vi "LightSensor.vi"() -> ()   [LabVIEW 2024]
uses:
  Driver/CTIPicoVISA.lvlib
panel:
  out "Identity":T1
  out "Value":u16(graph)
  in  "GroveConnector":enum16{"A0", "A1", "A2"}(ring)
  in  "stop":bool
  in  "VISA resource name in":refnum<visa-resource-name>="COM7"
  out "error out":errorcluster
  # "https://wiki.seeedstudio.com/Grove-Light_Sensor/#upgradable-to-industrial-sensors"
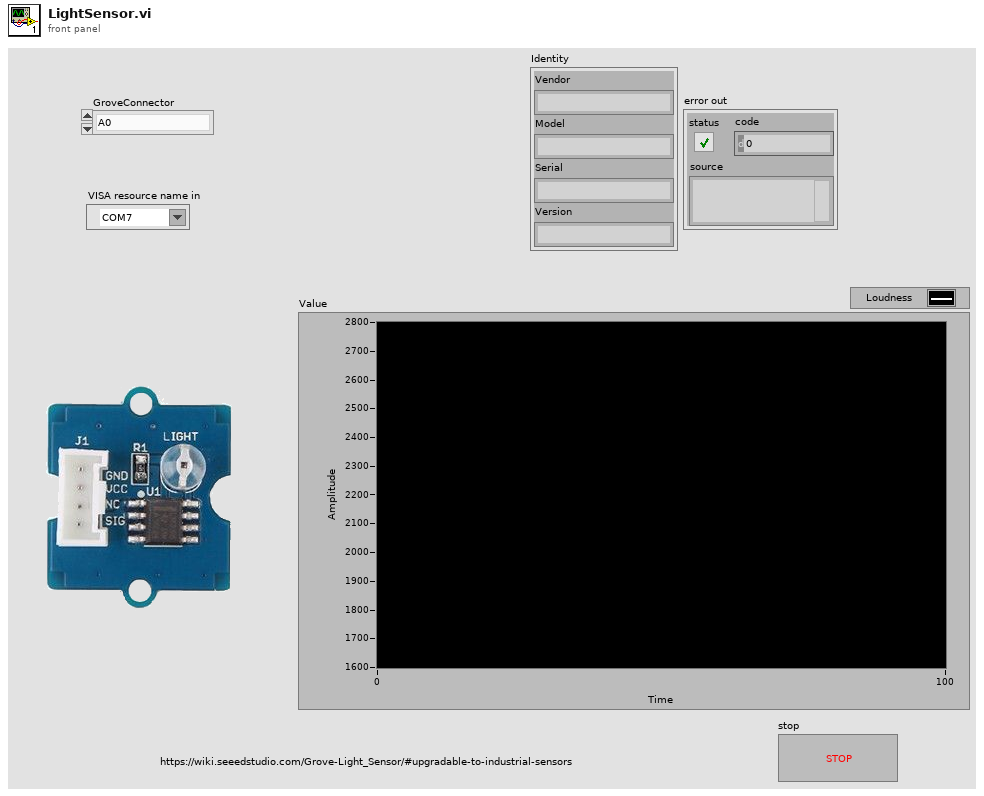
[diagram p1: front panel]
types:
  T1 = cluster{"Vendor":string, "Model":string, "Serial":string, "Version":string}
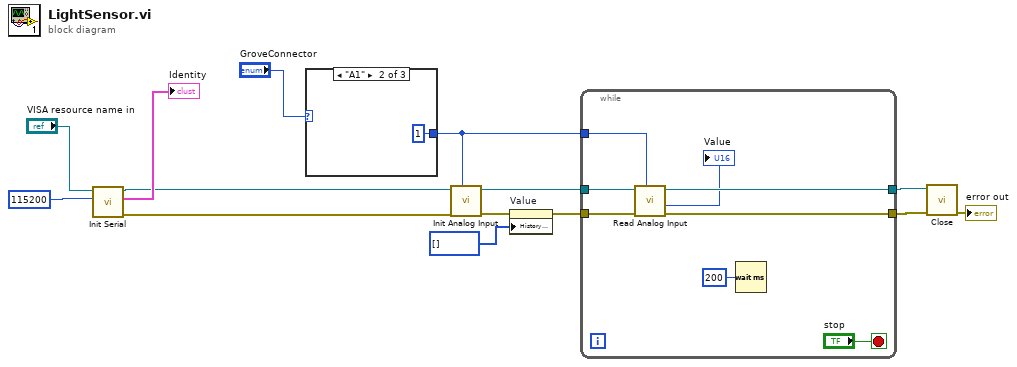
[diagram p0: block diagram]
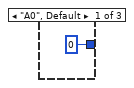
[diagram p2: hidden frame]
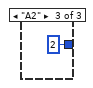
[diagram p3: hidden frame]
diagram:
  n1 = call "Init Serial.vi"("Baud (115200)"=u32 115200, "VISA resource name in"="VISA resource name in") -> ("error out"=w7:errorcluster, "Identity"=→"Identity":T1, "VISA resource name Out"=w8:refnum<visa-resource-name>)  [unwired: 7 in]
  n2 = case shown="\"A1\"" "GroveConnector" {
    tunnel: [0 ("GPIO") 1 ("GPIO") 2 ("GPIO")] -> w10
    frame "A0", Default {
    }
    frame "A1" {
    }
    frame "A2" {
    }
  }
  n3 = call "Init Analog Input.vi"("ADC"=w10, "error in (no error)"=w7, "VISA resource name in"=w8) -> ("error out"=w1:errorcluster, "VISA resource name"=w11:refnum<visa-resource-name>)  [unwired: 7 in]
  n4 = property on="Value" class="WFChart (strict)"(error in=w1, "History Data"=u16[] []) -> (error out=w2:errorcluster)  [unwired: 1 in, 1 out]
  n5 = while {
    tunnel: w11 -> [w23]
    tunnel: w10 -> [w22]
    tunnel: [w21] -> w6
    tunnel: [w19] -> w5
    tunnel: w2 -> [w24]
    stop <- "stop" stop-if-true
    n6 = call "Read Analog Input.vi"("ADC"=w22, "error in (no error)"=w24, "VISA resource name in"=w23) -> ("error out"=w19:errorcluster, "Value"=→"Value":u16, "VISA resource name"=w21:refnum<visa-resource-name>)  [unwired: 6 in]
    n7 = Wait (ms)(milliseconds to wait=u32 200) -> ()  [unwired: 1 out]
  }
  n8 = call "Close.vi"("error in (no error)"=w5, "VISA resource name in"=w6) -> ("error out"=→"error out":errorcluster)  [unwired: 9 in]
